vi "Compute.vi"(8 "error in (no error)":errorcluster, 9 "Data Channels":T4, 10 "x-var":T1, 11 "Normalize in":refnum<class "Normalize.lvclass">) -> (0 "error out":errorcluster, 1 "Add'l Data Channels":T4, 3 "Normalize out":refnum<class "Normalize.lvclass">)   [LabVIEW 2012, in "Normalize.lvclass"]
doc: "Given a data channel and an x-coordinate, compute and return one or more new data channels."
uses:
  Normalize.lvclass
  Instruments/Utility Classes/Readable/Data Channels.ctl
  Instruments/Utility Classes/Readable/Data Channel.ctl
  Instruments/Utility Classes/Readable/Data Point.ctl
  Instruments/Utility Classes/Readable/Time.ctl
  Instruments/Utility Classes/Readable/X.ctl
  Aux Data Source/Aux Data Source.lvclass
  Instruments/Utility Classes/Readable/Readable.lvclass
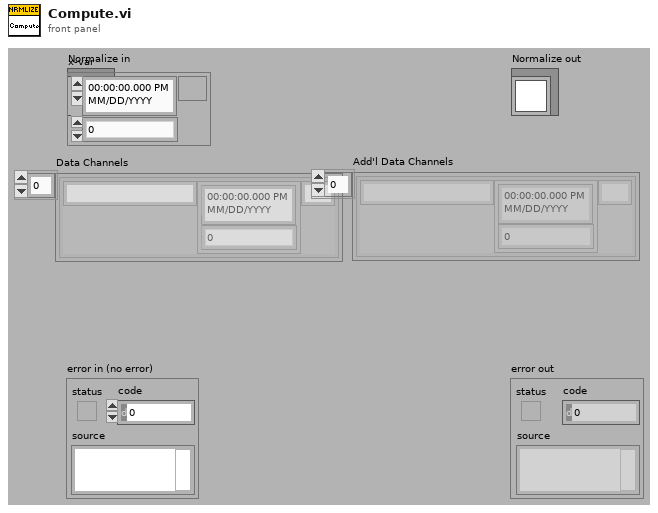
[diagram p1: front panel]
types:
  T1 = typedef "Readable.lvclass/Data Point.ctl" = cluster{"t":T2, "x":T3}
  T2 = typedef "Readable.lvclass/Time.ctl" = timestamp
  T3 = typedef "Readable.lvclass/X.ctl" = dbl
  T4 = typedef "Readable.lvclass/Data Channels.ctl" = T5[]
  T5 = typedef "Readable.lvclass/Data Channel.ctl" = cluster{"Name":string, "Data Point":T1, "Unit":string}
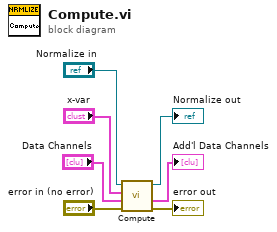
[diagram p0: block diagram]
diagram:
  n1 = call-parent "Compute.vi"("error in (no error)"="error in (no error)", "Data Channels"="Data Channels", "x-var"="x-var", "Aux Data Source in"="Normalize in") -> ("error out"=→"error out":errorcluster, "Add'l Data Channels"=→"Add'l Data Channels":T4, "Aux Data Source out"=→"Normalize out":refnum<class "Normalize.lvclass">)  [unwired: 5 in]
